vi "Stop Core.vi"(10 "final error code":i32, 11 "Actor_Autotest in":refnum<class "Actor_Autotest.lvclass">) -> (3 "Actor_Autotest out":refnum<class "Actor_Autotest.lvclass">)   [LabVIEW 2020, in "Library Core.lvlib" / "Actor_Autotest.lvlib" / "Actor_Autotest.lvclass"]
doc: "(<B>Filename</B>: Actor Framework.lvlib:Actor.lvclass:Stop Core.vi)\n\nDefines what the actor does before it stops. Use the <B>final error code</B> input to determine whether the actor shut down in response to an error.\n\nBy default, this method does nothing. A descendant class may override it to define behavior, such as shutting down any processes the actor initiated in its override of the Actor Core method."
uses:
  Actor_Autotest.lvclass
  Actor_Autotest.lvclass/Actor_Autotest.ctl
  <vilib>/ActorFramework/Actor/Actor.lvclass
  Commun VI/Library Commun.lvlib
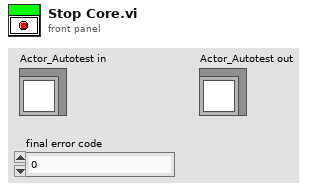
[diagram p1: front panel]
types:
  T1 = enum16{"Init", "Add Actor", "Delete Actor", "Get Actor Queue", "Get Log Actor Queue", "List all actors"}
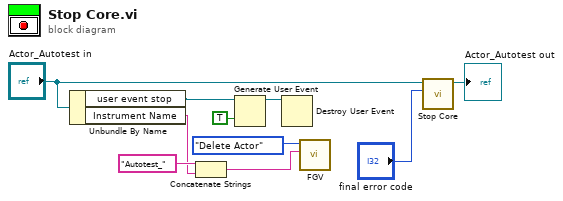
[diagram p0: block diagram]
diagram:
  n1 = Unbundle By Name("Actor_Autotest in") -> ("user event stop"=w8:refnum<user-event>, "Instrument Name"=w2:string)
  n2 = Concatenate Strings("Autotest_", w2) -> (w1:string)
  n3 = Generate User Event(user event=w8, event data cluster=TRUE ("event data")) -> (user event out=w6:refnum<user-event>)  [unwired: 2 in, 1 out]
  n4 = Destroy User Event(user event=w6) -> ()  [unwired: 1 in, 1 out]
  n5 = call "FGV.vi"("Actor name"=w1, "Action"=T1."Delete Actor") -> ()  [unwired: 7 in, 3 out]
  n6 = call-parent "Stop Core.vi"("final error code"="final error code", "Actor in"="Actor_Autotest in") -> ("Actor out"=→"Actor_Autotest out":refnum<class "Actor_Autotest.lvclass">)  [unwired: 9 in]
